vi "Вывод напряжения.vi"() -> ()   [LabVIEW 2017]
doc: "This VI is an exercise in the LabVIEW Basics I course."
panel:
  out "Выходное напряжение":dbl
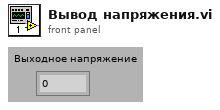
[diagram p1: front panel]
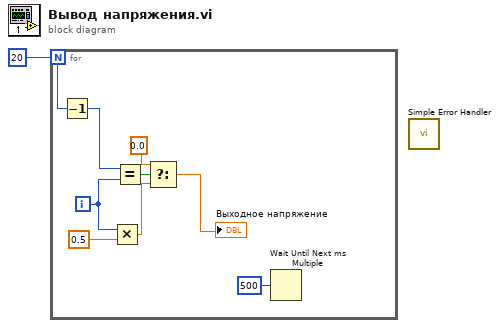
[diagram p0: block diagram]
diagram:
  n1 = for {
    N: 20 -> [w8]
    i -> [w6]
    n2 = Decrement(x=w8) -> (x-1=w5:i32)
    n3 = Multiply(x=w6, y=0.5) -> (x*y=w3:dbl)
    n4 = Equal?(x=w5, y=w6) -> (x = y?=w7:bool)
    n5 = Select(t=0.0, s=w7, f=w3) -> (s? t:f=→"Выходное напряжение":dbl)
    n6 = Wait Until Next ms Multiple(millisecond multiple=u32 500) -> ()  [unwired: 1 out]
  }
  n7 = call <vilib>:"Simple Error Handler.vi"() -> ()  [unwired: 5 in, 5 out]
